vi "Conductus Ramp Power.vi"(2 "Point #":i32, 4 "Parameters":dbl[](array[numeric]) format="%.3e", 5 "Instrument Address":refnum<visa-resource-name>) -> (0 "Stop":bool, 1 "Data Out":dbl[](array[numeric]) format="%.2e")   [LabVIEW 2019]
doc: "This VI reads the sample output of the Lakeshore DRC 93C or 82C temperature controller. The output is an array consisting of the single reading. The input is the numeric GPIB address.\nScott Hannahs, F. Bitter National Magnet Lab, 1993"
panel:
  # "Starting Power"
  # "Ending Power"
  # "Time (Min)"
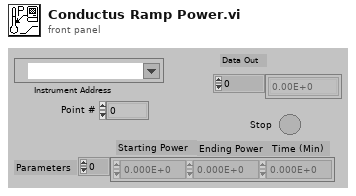
[diagram p1: front panel]
types:
  T1 = cluster{"Parameters[0]":dbl, "Parameters[1]":dbl, "Parameters[2]":dbl}
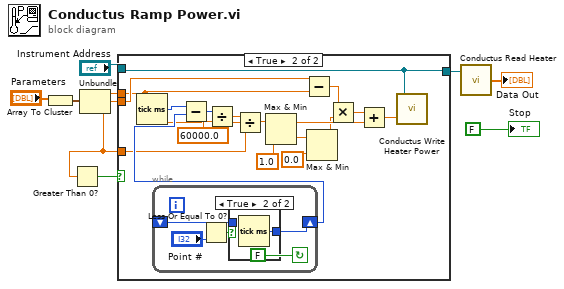
[diagram p0: block diagram]
diagram:
  n1 = Array To Cluster(array="Parameters") -> (cluster=w6:T1)
  n2 = Unbundle(w6) -> ("Parameters[0]"=w4:dbl, "Parameters[1]"=w5:dbl, "Parameters[2]"=w8:dbl)
  n3 = Greater Than 0?(x=w8) -> (x > 0?=w10:bool)
  n4 = case shown="True" w10 {
    tunnel: w8 -> [_ w23]
    tunnel: "Instrument Address" -> [w11 w12]
    tunnel: w5 -> [_ w18]
    tunnel: w4 -> [_ w17]
    tunnel: [w11 w12] -> w2
    frame False {
    }
    frame True {
      n5 = Tick Count (ms)() -> (millisecond timer value=w28:u32)
      n6 = while {
        shift-left: _ -> [w30]
        shift-right: [w31] -> w27
        stop <- FALSE continue-if-true
        n7 = Less Or Equal To 0?(x="Point #") -> (x <= 0?=w32:bool)
        n8 = case shown="True" w32 {
          tunnel: [w34 w35] -> w31
          tunnel: w30 -> [w34 _]
          frame False {
          }
          frame True {
            n9 = Tick Count (ms)() -> (millisecond timer value=w35:u32)
          }
        }
      }
      n10 = Subtract(x=w28, y=w27) -> (x-y=w26:u32)
      n11 = Divide(x=w26, y=60000.0) -> (x/y=w24:dbl)
      n12 = Divide(x=w24, y=w23) -> (x/y=w21:dbl)
      n13 = Max & Min(x=w21, y=1.0) -> (min(x,y)=w14:dbl)  [unwired: 1 out]
      n14 = Subtract(x=w18, y=w17) -> (x-y=w22:dbl)
      n15 = Max & Min(x=w14, y=0.0) -> (max(x,y)=w15:dbl)  [unwired: 1 out]
      n16 = Multiply(x=w22, y=w15) -> (x*y=w20:dbl)
      n17 = Add(x=w20, y=w17) -> (x+y=w13:dbl)
      n18 = call "Conductus Write Heater Power.vi"("Setpoint"=w13, "Instrument Address"=w12) -> ()  [unwired: 1 in]
    }
  }
  n19 = call "Conductus Read Heater.vi"("Instrument Address"=w2) -> ("Heater Power %"=→"Data Out":dbl[])
  "Stop" <- FALSE
